vi "OperationCall.vi"(0 "Arithmetic in":refnum<class "Arithmetic.lvclass">, 5 "Sub Panel":refnum<vi>, 7 "user event out":refnum<user-event>, 9 "event source":refnum<user-event>, 11 "error in (no error)":errorcluster) -> (4 "Arithmetic out":refnum<class "Arithmetic.lvclass">, 15 "error out":errorcluster)   [LabVIEW 2023, in "Arithmetic.lvclass"]
uses:
  Arithmetic.lvclass
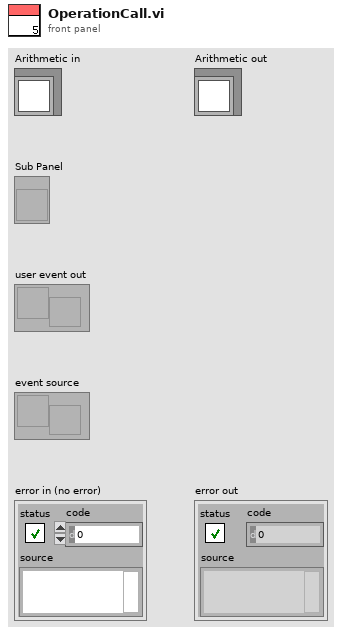
[diagram p1: front panel]
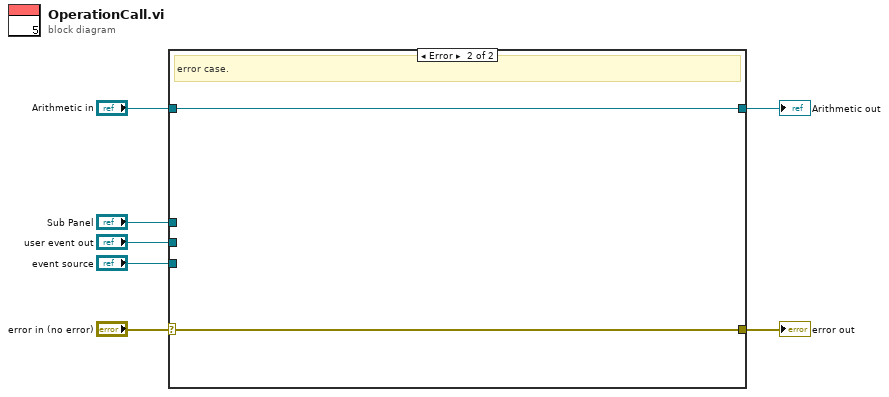
[diagram p0: block diagram]
diagram:
  n1 = case shown="Error" "error in (no error)" {
    selector: "error in (no error)" -> [w8 w11]
    tunnel: [w8 w11] -> w6
    tunnel: [w9 w10] -> w4
    tunnel: "Arithmetic in" -> [w9 w10]
    tunnel: "Sub Panel" -> [_ _]
    tunnel: "user event out" -> [_ _]
    tunnel: "event source" -> [_ _]
    frame No Error {
      # "Wire the error cluster across even in the \"No Error\"\ncase so that warnings get propagated."
      # "No error case."
    }
    frame Error {
      # "error case."
    }
  }
  "error out" <- w6
  "Arithmetic out" <- w4
